vi "Read Module type.vi"(8 "error in (no error)":errorcluster, 11 "Start-module in":refnum<class "Start-client.lvclass">) -> (0 "error out":errorcluster, 2 "Module type":string, 3 "Start-module out":refnum<class "Start-client.lvclass">)   [LabVIEW 2013, in "SLMAPI.lvlib" / "Start-client.lvclass"]
uses:
  Start-client.lvclass
  Start-client.lvclass/Start-client.ctl
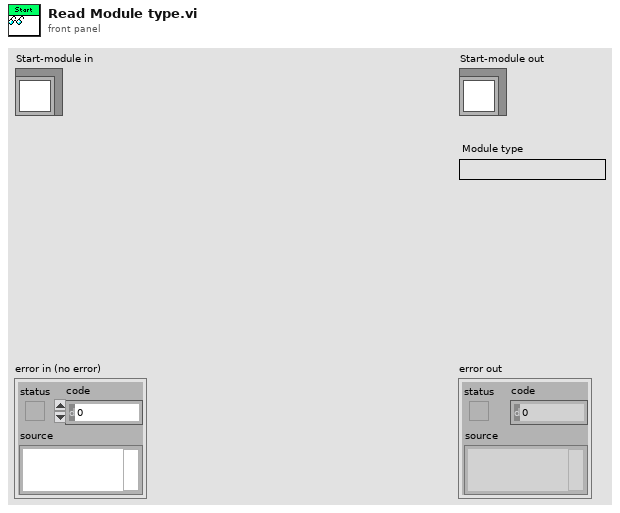
[diagram p1: front panel]
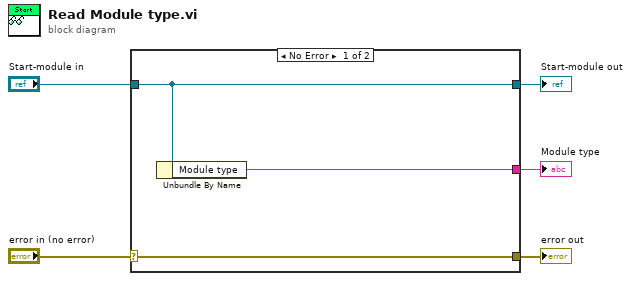
[diagram p0: block diagram]
diagram:
  n1 = case shown="No Error" "error in (no error)" {
    selector: "error in (no error)" -> [w8 w9]
    tunnel: [w8 w9] -> w4
    tunnel: [w7 w10] -> w2
    tunnel: "Start-module in" -> [w7 w10]
    tunnel: [w6 _] -> w1
    frame No Error {
      n2 = Unbundle By Name(w7) -> ("Module type"=w6:string)
    }
    frame Error {
    }
  }
  "error out" <- w4
  "Start-module out" <- w2
  "Module type" <- w1
